vi "Intake Controller.vi"(8 "error in":errorcluster) -> ()   [LabVIEW 2016]
doc: "This VI executes continuously carrying out the current operation and responding to updates or new operations. It will often contain the timing or control code that is difficult to place directly in TeleOp. This VI generally opens all sensors and motors and isolates the rest of the robot code from knowing how the operations are carried out."
uses:
  Intake Setpoints.ctl
  Intake Operations.ctl
  <vilib>/Rock Robotics/SystemInterfaces/DIO/FPGA_DIOPWMChannel.ctl
  <vilib>/Rock Robotics/WPI/MotorControl/WPI_MotorControlOpen SPARK.vi
  <vilib>/Rock Robotics/Network Tables/NT Write Boolean.vi
panel:
  out "Current\nCmd":string
  # "Tip: It may be helpful to observe inputs and sensor values.\nYou may also want to display tuning or debugging controls."
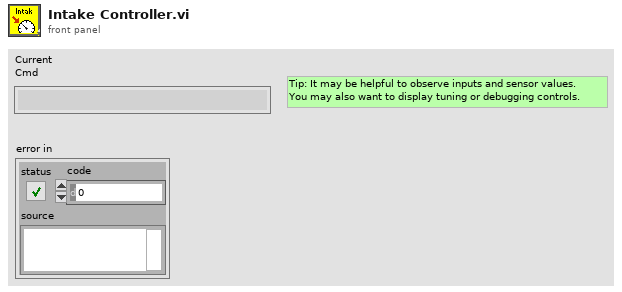
[diagram p1: front panel]
types:
  T1 = typedef "FPGA_DIOPWMChannel.ctl" = enum8{"PWM 0", "PWM 1", "PWM 2", "PWM 3", "PWM 4", "PWM 5", "PWM 6", "PWM 7", "PWM 8", "PWM 9", "PWM MXP 0", "PWM MXP 1", "PWM MXP 2", "PWM MXP 3", "PWM MXP 4", "PWM MXP 5", "PWM MXP 6", "PWM MXP 7", "PWM MXP 8", "PWM MXP 9", "Invalid"}
  T2 = typedef "Intake Setpoints.ctl" = cluster{"Operation":T3, "Setpoint":dbl, "Duration":dbl}
  T3 = typedef "Intake Operations.ctl" = enum16{"Reserve", "Read Current", "Immediate"}
  T4 = typedef "WPI_MotorControlDeviceRef.ctl" = cluster{"DeviceStatus":errorcluster, "Type":T5, "PWM":cluster{"PWM Channel":T1, "DeadBand":T6}, "CAN":cluster{"Device Number":u8, "SetOutput VI Ref":variant, "GetOutput VI Ref":variant, "Enable VI Ref":variant, "Disable VI Ref":variant, "Data":variant}, "Invert":bool}
  T5 = typedef "WPI_MotorControlType.ctl" = enum16{"PWM", "CAN"}
  T6 = typedef "WPI_PWMDeadband.ctl" = cluster{"Name":string, "maxPositivePwm":i32, "minPositivePwm":i32, "centerPwm":i32, "maxNegativePwm":i32, "minNegativePwm":i32, "angularRange":u16}
  T7 = typedef "Command Status Info.ctl" = cluster{"Name":string, "Status":T8, "notifier out":T9}
  T8 = typedef "Completion Status.ctl" = enum16{"Successful", "Aborted", "Incomplete"}
  T9 = typedef "Completion Notifier.ctl" = refnum<notifier>
  T10 = cluster{"Default Command":T2, "Command Timing":cluster{"Start Time (ms)":u32, "Iterations":i32}, "Command Arguments":cluster{"Command Info":T7, "Description":string, "Default Command":T2, "notifier out":refnum<notifier>, "Subsystem Name":string}}
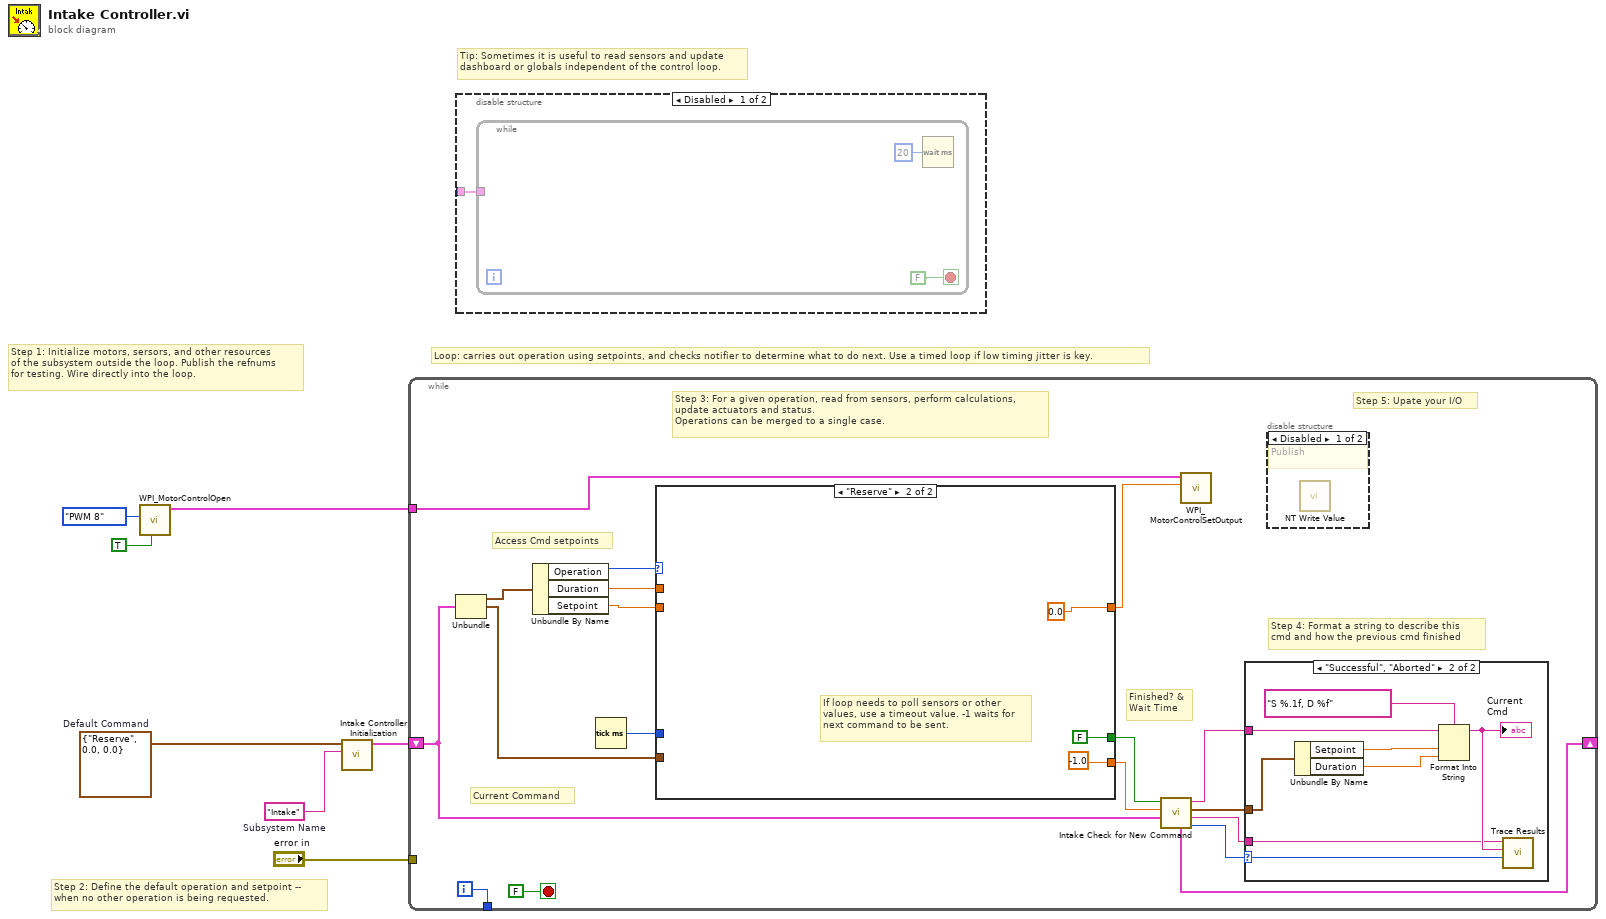
[diagram p0: block diagram]
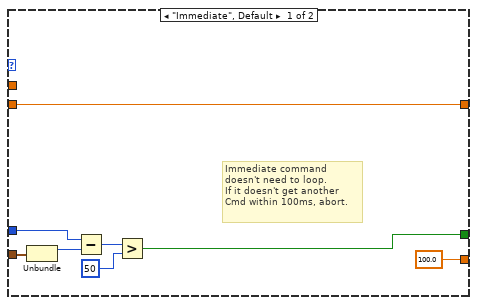
[diagram p5: hidden frame]
diagram:
  w4 = T2 {"Operation"=enum."Reserve", "Setpoint"=0.0, "Duration"=0.0}  # Default Command
  w5 = "Intake"  # Subsystem Name
  # "Tip: Sometimes it is useful to read sensors and update\ndashboard or globals independent of the control loop."
  # "Step 2: Define the default operation and setpoint --\nwhen no other operation is being requested."
  # "Step 1: Initialize motors, sersors, and other resources\nof the subsystem outside the loop. Publish the refnums\nfor testing. Wire directly into the loop."
  # "Loop: carries out operation using setpoints, and checks notifier to determine what to do next. Use a timed loop if low timing jitter is key."
  n1 = call-poly <vilib>:"WPI_MotorControlOpen.vi"("Invert"=TRUE, "PWM Channel"=FPGA_DIOPWMChannel."PWM 8") -> ("MotorControlDeviceRef"=w2:T4)  [unwired: 8 in, 1 out]
  n2 = call "Intake Controller Initialization.vi"("Subsystem Name"=w5, "Default Command"=w4) -> ("Command Info"=w6:T10)  [unwired: 9 in]
  n3 = while {
    shift-right: [w16] -> _
    shift-left: w6 -> [w17]
    tunnel: [w24] -> _
    tunnel: "error in" -> [_]
    tunnel: w2 -> [w9]
    i -> [w24]
    stop <- FALSE stop-if-true
    # "Step 5: Upate your I/O"
    # "Step 4: Format a string to describe this\ncmd and how the previous cmd finished"
    # "Current Command"
    # "Access Cmd setpoints"
    # "Finished? &\nWait Time"
    # "Step 3: For a given operation, read from sensors, perform calculations,\nupdate actuators and status.\nOperations can be merged to a single case."
    n4 = Unbundle(w17) -> ("Default Command"=w23:T2, "Command Timing"=w19:cluster{"Start Time (ms)":u32, "Iterations":i32})  [unwired: 1 out]
    n5 = Unbundle By Name(w23) -> ("Operation"=w22:T3, "Duration"=w21:dbl, "Setpoint"=w18:dbl)
    n6 = Tick Count (ms)() -> (millisecond timer value=w20:u32)
    n7 = case shown="\"Reserve\"" w22 {
      tunnel: [100.0 -1.0] -> w14
      tunnel: [w35 FALSE ("ignore previous (F)")] -> w15
      tunnel: w19 -> [w37 _]
      tunnel: w21 -> [_ _]
      tunnel: w20 -> [w36 _]
      tunnel: w18 -> [w34 _]
      tunnel: [w34 0.0] -> w8
      frame "Immediate", Default {
        # "Immediate command\ndoesn't need to loop.\nIf it doesn't get another\nCmd within 100ms, abort."
        n8 = Unbundle(w37) -> ("Start Time (ms)"=w40:u32)  [unwired: 1 out]
        n9 = Subtract(x=w36, y=w40) -> (x-y=w39:u32)
        n10 = Greater?(x=w39, y=u8 50 ("Left Motor")) -> (0:w35:bool)
      }
      frame "Reserve" {
        # "If loop needs to poll sensors or other\nvalues, use a timeout value. -1 waits for\nnext command to be sent."
      }
    }
    n11 = call "Intake Check for New Command.vi"("Current Command"=w17, "Wait time (ms)"=w14, "Finished?"=w15) -> ("Completion"=w10:T8, "Subsystem Name"=w11:string, "Current Command"=w12:T2, "Initial Trace String"=w13:string, "NextCommand"=w16:T10)  [unwired: 4 in]
    n12 = call <vilib>:"WPI_MotorControlSetOutput.vi"("Output"=w8, "MotorControlDevRef"=w9) -> ()  [unwired: 7 in, 3 out]
    n13 = case shown="\"Successful\", \"Aborted\"" w10 {
      selector: w10 -> [_ w33]
      tunnel: w13 -> [_ w29]
      tunnel: w12 -> [_ w30]
      tunnel: w11 -> [_ w26]
      frame "Incomplete", Default {
        # "Continuing current command"
      }
      frame "Successful", "Aborted" {
        # "Report and setup for next command"
        n14 = Unbundle By Name(w30) -> ("Setpoint"=w32:dbl, "Duration"=w27:dbl)
        n15 = Format Into String(format string="S %.1f, D %f", initial string=w29, w32, w27) -> (resulting string=w28:string)  [unwired: 1 in, 1 out]
        "Current\nCmd" <- w28
        n16 = call <vilib>:"Trace Results.vi"("Status of previous command"=w33, "Description"=w28, "Subsystem"=w26) -> ()  [unwired: 9 in]
      }
    }
    n17 = disable-structure shown="Disabled" {
      frame Disabled {
        # "Publish"
        n18 = call-poly <vilib>:"NT Write Value.vi"() -> ()  [unwired: 11 in, 1 out]
      }
      frame Enabled {
      }
    }
  }
  n19 = disable-structure shown="Disabled" {
    disable-tunnel: _ -> [w45 _]
    frame Disabled {
      n20 = while {
        tunnel: w45 -> [_]
        stop <- FALSE stop-if-true
        n21 = Wait (ms)(milliseconds to wait=u32 20) -> ()  [unwired: 1 out]
      }
    }
    frame Enabled {
    }
  }
